vi "GAMBAR.vi"() -> ()   [LabVIEW 2024]
panel:
  out "new picture":picture
  in  "?":path
  in  "Ring":u16(ring) items=["PNG"=2, "JPEG"=1]
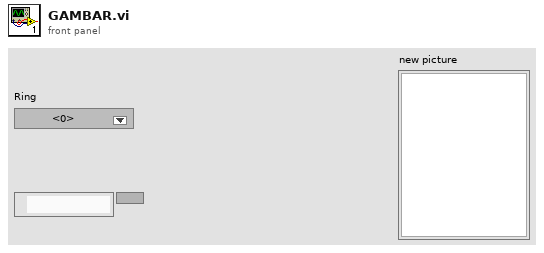
[diagram p1: front panel]
types:
  T1 = typedef "imagedata.ctl" = cluster{"image type":i32, "image depth":i32, "image":u8[], "mask":u8[], "colors":u32[], "Rectangle":cluster{"left":i16, "top":i16, "right":i16, "bottom":i16}}
  T2 = typedef "LVBoundsTypeDef.ctl" = cluster{"Width":u32, "Height":u32}
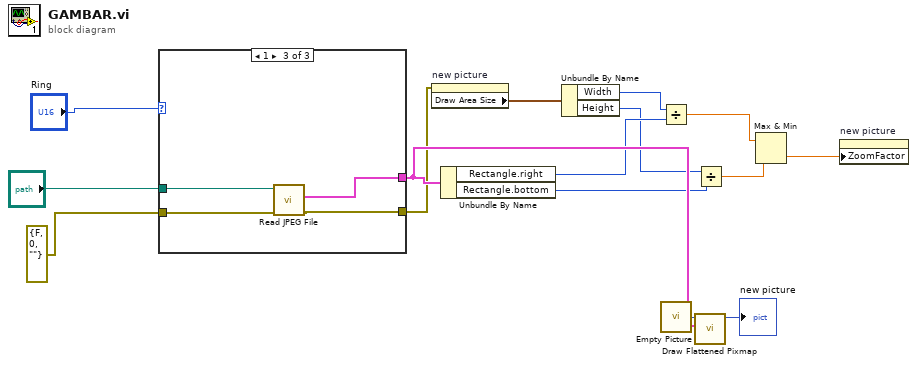
[diagram p0: block diagram]
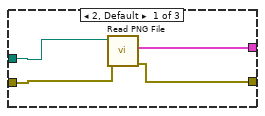
[diagram p2: hidden frame]
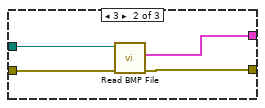
[diagram p3: hidden frame]
diagram:
  n1 = case shown="1" "Ring" {
    tunnel: errorcluster {"status"=FALSE, "code"=0, "source"=""} ("error constant") -> [w19 w23 w27]
    tunnel: [w18 w22 w26] -> w9
    tunnel: "?" -> [w17 w21 w25]
    tunnel: [w16 w20 w24] -> w10
    frame 2, Default {
      n2 = call <vilib>:"Read PNG File.vi"("error in (no error)"=w19, "path to PNG file"=w17) -> ("error out"=w18:errorcluster, "image data"=w16:T1)  [unwired: 7 in, 1 out]
    }
    frame 3 {
      n3 = call <vilib>:"Read BMP File.vi"("error in (no error)"=w23, "path to BMP file"=w21) -> ("error out"=w22:errorcluster, "image data"=w20:T1)  [unwired: 7 in, 1 out]
    }
    frame 1 {
      n4 = call <vilib>:"Read JPEG File.vi"("error in (no error)"=w27, "path to JPEG file"=w25) -> ("error out"=w26:errorcluster, "image data"=w24:T1)  [unwired: 7 in, 1 out]
    }
  }
  n5 = property on="new picture" class="Pict"(error in=w9) -> ("Draw Area Size"=w8:T2)  [unwired: 1 in, 2 out]
  n6 = Unbundle By Name(w10) -> ("Rectangle.right"=w6:i16, "Rectangle.bottom"=w4:i16)
  n7 = Unbundle By Name(w8) -> ("Width"=w7:u32, "Height"=w5:u32)
  n8 = Divide(x=w7, y=w6) -> (x/y=w3:dbl)
  n9 = call "Empty Picture"() -> ("empty picture"=w11:picture)
  n10 = call <vilib>:"Draw Flattened Pixmap.vi"("image data"=w10, "picture"=w11) -> ("new picture"=→"new picture":picture)  [unwired: 7 in]
  n11 = Divide(x=w5, y=w4) -> (x/y=w2:dbl)
  n12 = Max & Min(x=w3, y=w2) -> (min(x,y)=w1:dbl)  [unwired: 1 out]
  n13 = property on="new picture" class="Pict"("ZoomFactor"=w1) -> ()  [unwired: 2 in, 2 out]
